vi "Parse Value.vi"(8 "error in (no error)":errorcluster, 10 "Index In":i32, 11 "JSON String":string) -> (0 "error out":errorcluster, 2 "Index Out":i32, 3 "JSON Value out":refnum<class "JSON Value.lvclass">)   [LabVIEW 2016, in "JSON Value.lvclass"]
uses:
  JSON Value.lvclass
  subVIs/Errors.ctl
  New JSON Value/New JSON (Null).vi
  New JSON Value/New JSON (Boolean).vi
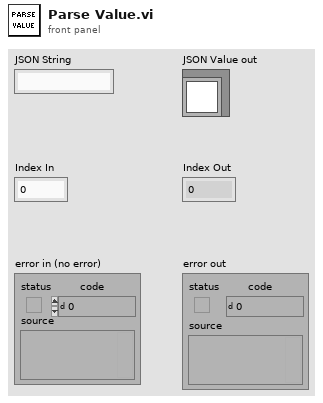
[diagram p1: front panel]
types:
  T1 = typedef "JSON Value.lvclass/Errors.ctl" = enum8{"No key", "Key path type", "Array OOB", "Type Mismatch", "Invalid Token"}
  T2 = typedef "JSON Value.lvclass/Token Type.ctl" = enum8{"NONE", "CURLY_OPEN", "CURLY_CLOSE", "SQUARED_OPEN", "SQUARED_CLOSE", "COLON", "COMMA", "STRING", "NUMBER", "TRUE", "FALSE", "NULL"}
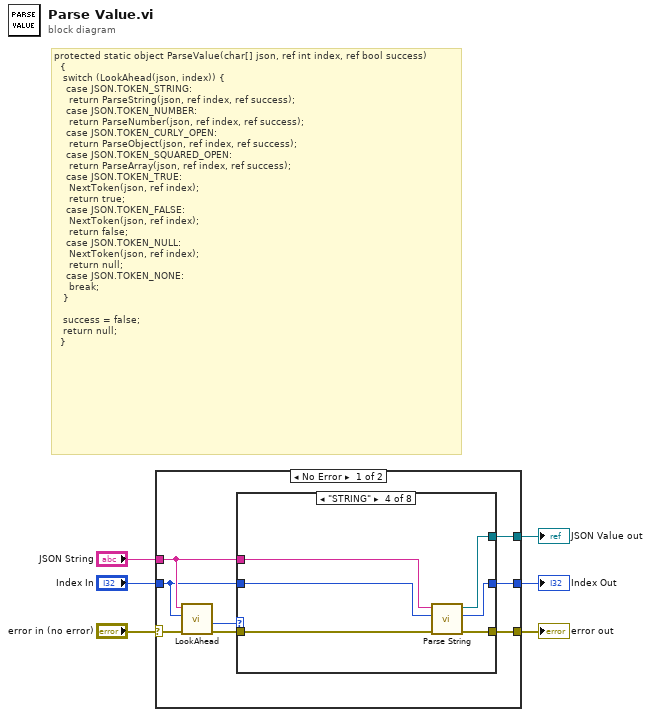
[diagram p0: block diagram]
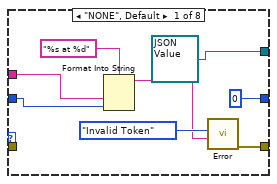
[diagram p2: hidden frame]
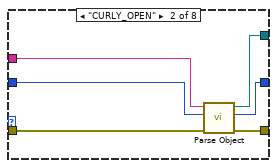
[diagram p3: hidden frame]
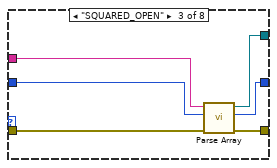
[diagram p4: hidden frame]
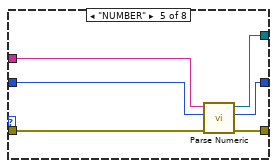
[diagram p5: hidden frame]
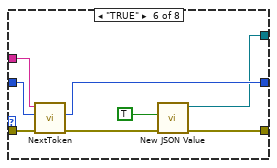
[diagram p6: hidden frame]
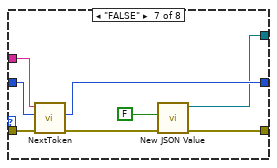
[diagram p7: hidden frame]
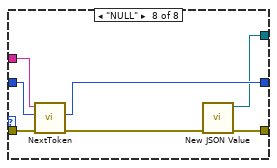
[diagram p8: hidden frame]
diagram:
  # "protected static object ParseValue(char[] json, ref int index, ref bool success)\n\t\t{\n\t\t\tswitch (LookAhead(json, index)) {\n\t\t\t\tcase JSON.TOKEN_STRING:\n\t\t\t\t\treturn ParseString(json, ref index, ref success);\n\t\t\t\tcase JSON.TOKEN_NUMBER:\n\t\t\t\t\treturn ParseNumber(json, ref index, ref success);\n\t\t\t\tcase JSON.TOKEN_CURLY_OPEN:\n\t\t\t\t\treturn ParseObject(json, ref index, ref success);\n\t\t\t\tcase JSON.TOKEN_SQUARED_OPEN:\n\t\t\t\t\treturn ParseArray(json, ref index, ref success);\n\t\t\t\tcase JSON.TOKEN_TRUE:\n\t\t\t\t\tNextToken(json, ref index);\n\t\t\t\t\treturn true;\n\t\t\t\tcase JSON.TOKEN_FALSE:\n\t\t\t\t\tNextToken(json, ref index);\n\t\t\t\t\treturn false;\n\t\t\t\tcase JSON.TOKEN_NULL:\n\t\t\t\t\tNextToken(json, ref index);\n\t\t\t\t\treturn null;\n\t\t\t\tcase JSON.TOKEN_NONE:\n\t\t\t\t\tbreak;\n\t\t\t}\n\n\t\t\tsuccess = false;\n\t\t\treturn null;\n\t\t}"
  n1 = case shown="No Error" "error in (no error)" {
    selector: "error in (no error)" -> [w14 w70]
    tunnel: [w12 w70] -> w5
    tunnel: "JSON String" -> [w8 _]
    tunnel: "Index In" -> [w7 _]
    tunnel: [w10 _] -> w1
    tunnel: [w9 _] -> w2
    frame No Error {
      n2 = call "LookAhead.vi"("error in (no error)"=w14, "Index"=w7, "JSON String"=w8) -> ("error out"=w13:errorcluster, "TOKEN"=w11:T2)  [unwired: 7 in]
      n3 = case shown="\"STRING\"" w11 {
        tunnel: w13 -> [_ w26 w32 w38 w44 w51 w60 w66]
        tunnel: [w21 w25 w31 w37 w43 w48 w57 w64] -> w12
        tunnel: [refnum<class "JSON Value.lvclass"> refnum ("JSON Object in") w23 w29 w35 w41 w47 w55 w63] -> w10
        tunnel: w8 -> [w18 w27 w34 w40 w46 w54 w58 w68]
        tunnel: w7 -> [w17 w28 w33 w39 w45 w53 w59 w67]
        tunnel: [0 ("Index Out") w24 w30 w36 w42 w52 w61 w65] -> w9
        frame "NONE", Default {
          n4 = Format Into String(format string="%s at %d", w18, w17) -> (resulting string=w16:string)  [unwired: 2 in, 1 out]
          n5 = call "Error.vi"("Data"=w16, "Error"=Errors."Invalid Token") -> ("error out"=w21:errorcluster)  [unwired: 8 in]
        }
        frame "CURLY_OPEN" {
          n6 = call "Parse Object.vi"("error in (no error)"=w26, "Index In"=w28, "JSON String"=w27) -> ("error out"=w25:errorcluster, "Index Out"=w24:i32, "JSON Value out"=w23:refnum<class "JSON Value.lvclass">)  [unwired: 6 in]
        }
        frame "SQUARED_OPEN" {
          n7 = call "Parse Array.vi"("error in (no error)"=w32, "Index In"=w33, "JSON String"=w34) -> ("error out"=w31:errorcluster, "Index Out"=w30:i32, "JSON Value out"=w29:refnum<class "JSON Value.lvclass">)  [unwired: 6 in]
        }
        frame "STRING" {
          n8 = call "Parse String.vi"("error in (no error)"=w38, "Index In"=w39, "JSON String"=w40) -> ("error out"=w37:errorcluster, "Index Out"=w36:i32, "JSON Value out"=w35:refnum<class "JSON Value.lvclass">)  [unwired: 5 in, 1 out]
        }
        frame "NUMBER" {
          n9 = call "Parse Numeric.vi"("error in (no error)"=w44, "Index In"=w45, "JSON String"=w46) -> ("error out"=w43:errorcluster, "Index Out"=w42:i32, "JSON Value out"=w41:refnum<class "JSON Value.lvclass">)  [unwired: 6 in]
        }
        frame "TRUE" {
          n10 = call "NextToken.vi"("error in (no error)"=w51, "Index In"=w53, "JSON String"=w54) -> ("error out"=w49:errorcluster, "Index Out"=w52:i32)  [unwired: 6 in, 1 out]
          n11 = call-poly "New JSON Value.vi"("error in (no error)"=w49, "value"=TRUE) -> ("error out"=w48:errorcluster, "JSON Value out"=w47:refnum<class "JSON Value.lvclass">)  [unwired: 8 in]
        }
        frame "FALSE" {
          n12 = call "NextToken.vi"("error in (no error)"=w60, "Index In"=w59, "JSON String"=w58) -> ("error out"=w62:errorcluster, "Index Out"=w61:i32)  [unwired: 6 in, 1 out]
          n13 = call-poly "New JSON Value.vi"("error in (no error)"=w62, "value"=FALSE) -> ("error out"=w57:errorcluster, "JSON Value out"=w55:refnum<class "JSON Value.lvclass">)  [unwired: 8 in]
        }
        frame "NULL" {
          n14 = call "NextToken.vi"("error in (no error)"=w66, "Index In"=w67, "JSON String"=w68) -> ("error out"=w69:errorcluster, "Index Out"=w65:i32)  [unwired: 6 in, 1 out]
          n15 = call-poly "New JSON Value.vi"("error in (no error)"=w69) -> ("error out"=w64:errorcluster, "JSON Value out"=w63:refnum<class "JSON Value.lvclass">)  [unwired: 9 in]
        }
      }
    }
    frame Error {
    }
  }
  "error out" <- w5
  "Index Out" <- w2
  "JSON Value out" <- w1
